vi "53 Invoke.vi"() -> ()   [LabVIEW 2020]
uses:
  _Subs/OpenDiagram/Open_XControl.xctl
panel:
  in  "OpenDiag":refnum<vi>(xcontrol)
  in  "Stop Button":bool
  in  "Excel":bool
  out "Waveform Chart":dbl(graph)
  # "03 Invoke example\nThis code takes the value of the Slide and adds it to the Gauge\n\nInstructions:\n1. Hit the Run arrow and after you have some data on the plot - port into Excel"
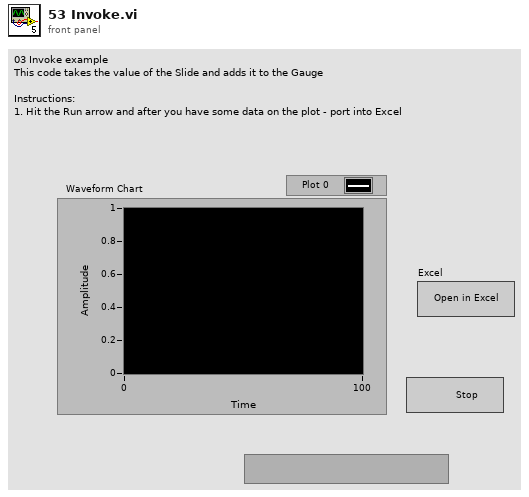
[diagram p1: front panel]
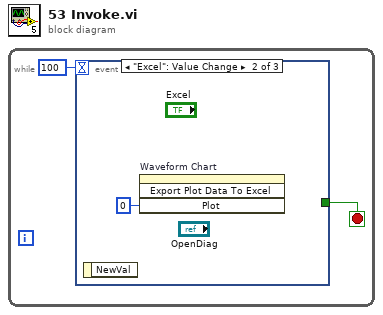
[diagram p0: block diagram]
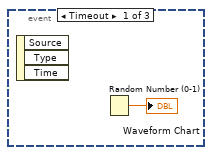
[diagram p2: hidden frame]
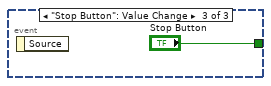
[diagram p3: hidden frame]
diagram:
  n1 = while {
    stop <- w1 stop-if-true
    n2 = event shown="[1] \"Excel\": Value Change" {
      selector: _ -> [_ _ _]
      dyn-events: _ -> [_ _ _]
      timeout: 100 -> [_ _ _]
      tunnel: [_ _ "Stop Button"] -> w1
      event Timeout {
        n3 = event-data() -> ()  [unwired: 1 in, 3 out]
        n4 = Random Number (0-1)() -> (number: 0 to 1=→"Waveform Chart":dbl)
      }
      event "Excel": Value Change {
        n5 = event-data() -> ()  [unwired: 1 in, 1 out]
        n6 = invoke on="Waveform Chart" class="WFChart (strict)" method="Export Plot Data To Excel"("Plot"=0) -> ()  [unwired: 3 in, 4 out]
      }
      event "Stop Button": Value Change {
        n7 = event-data() -> ()  [unwired: 1 in, 1 out]
      }
    }
  }
